vi "Analog Comparison.vi"(0 "Level":dbl, 2 "Condition":T1(ring), 5 "Data":dbl, 11 "error in":errorcluster) -> (4 "Result":bool, 15 "error out":errorcluster)   [LabVIEW 2010]
doc: "This VI does basic analog comparisons on the Data input."
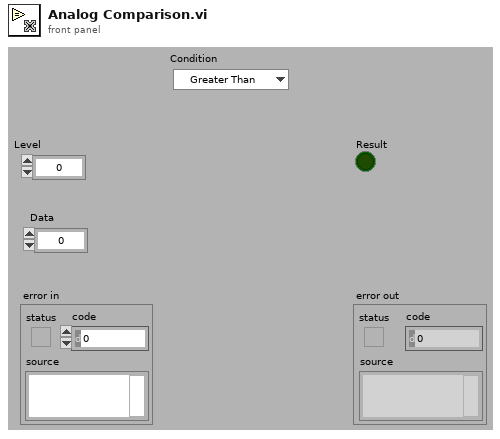
[diagram p1: front panel]
types:
  T1 = enum16{"Greater Than", "Greater Than or Equal", "Equal", "Not Equal", "Less Than", "Less Than or Equal"}
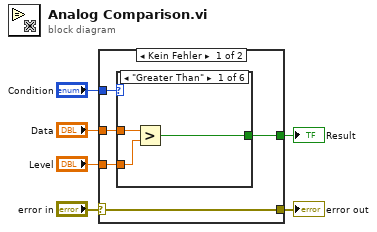
[diagram p0: block diagram]
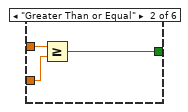
[diagram p2: hidden frame]
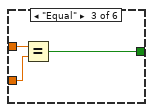
[diagram p3: hidden frame]
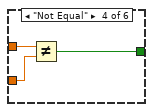
[diagram p4: hidden frame]
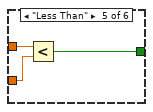
[diagram p5: hidden frame]
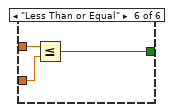
[diagram p6: hidden frame]
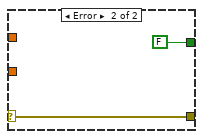
[diagram p7: hidden frame]
diagram:
  n1 = case shown="Kein Fehler" "error in" {
    selector: "error in" -> [w11 w31]
    tunnel: [w11 w31] -> w5
    tunnel: "Condition" -> [w10 _]
    tunnel: "Data" -> [w9 _]
    tunnel: "Level" -> [w8 _]
    tunnel: [w7 FALSE] -> w1
    frame No Error {
      n2 = case shown="\"Greater Than\"" w10 {
        tunnel: w9 -> [w14 w17 w20 w23 w26 w29]
        tunnel: w8 -> [w13 w16 w19 w22 w25 w28]
        tunnel: [w12 w15 w18 w21 w24 w27] -> w7
        frame "Greater Than" {
          n3 = Greater?(x=w14, y=w13) -> (0:w12:bool)
        }
        frame "Greater Than or Equal" {
          n4 = Greater Or Equal?(x=w17, y=w16) -> (x >= y?=w15:bool)
        }
        frame "Equal" {
          n5 = Equal?(x=w20, y=w19) -> (x = y?=w18:bool)
        }
        frame "Not Equal" {
          n6 = Not Equal?(x=w23, y=w22) -> (x != y?=w21:bool)
        }
        frame "Less Than" {
          n7 = Less?(x=w26, y=w25) -> (x < y?=w24:bool)
        }
        frame "Less Than or Equal" {
          n8 = Less Or Equal?(x=w29, y=w28) -> (x <= y?=w27:bool)
        }
      }
    }
    frame Error {
    }
  }
  "error out" <- w5
  "Result" <- w1
